vi "Set Crop Mode.vi"(8 "error in (no error)":errorcluster, 9 "reserved":i32, 10 "cropHeight":i32, 11 "active":i32) -> (0 "error out":errorcluster, 3 "function return":u32)   [LabVIEW 2014, in "atmcd32d.lvlib"]
doc: "unsigned int WINAPI SetCropMode(int active, int cropHeight, int reserved);"
uses:
  atmcd32d.lvlib
  atmcd32d.dll
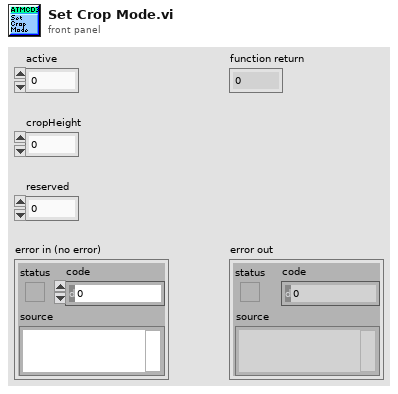
[diagram p1: front panel]
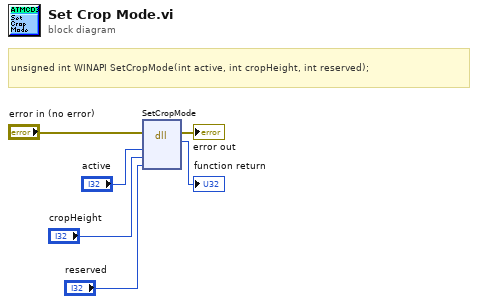
[diagram p0: block diagram]
diagram:
  # "unsigned int WINAPI SetCropMode(int active, int cropHeight, int reserved);"
  n1 = dll-call lib="C:/Users/Bakir/Documents/Lambda2-Testing/lib/Andorlib/atmcd32d.*" fn="SetCropMode"(error in="error in (no error)", "active"="active", "cropHeight"="cropHeight", "reserved"="reserved") -> (error out=→"error out":errorcluster, →"function return":u32)  [unwired: 5 in, 1 out]
